vi "ScanBasic.vi"(8 "error in (no error)":errorcluster, 11 "data":variant[][](array[variant])) -> (0 "error out":errorcluster, 3 "Array":T1[](array[typedef]))   [LabVIEW 2017, in "Client.lvlib" / "ParserSorter.lvlib"]
doc: "Perform Basic Parsing"
uses:
  ParserSorter.lvlib
  SR Data.ctl
  AE Group.ctl
  SR Status.ctl
  SR Level.ctl
  SR Type.ctl
  <vilib>/addons/database/_DB Variant To Data/Database Variant To Data.xnode
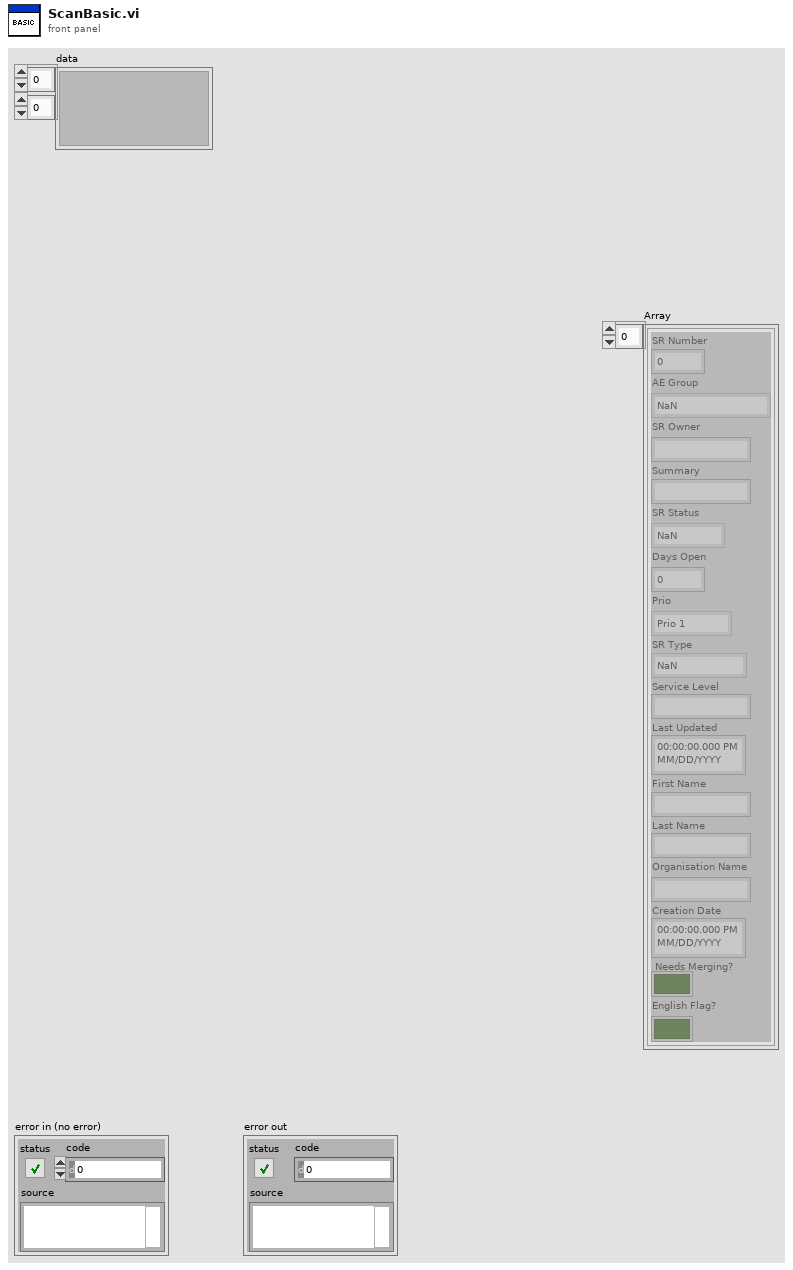
[diagram p1: front panel]
types:
  T1 = typedef "Client.lvlib/ParserSorter.lvlib/SR Data.ctl" = cluster{"SR Number":i64, "AE Group":T2, "SR Owner":string, "Summary":string, "SR Status":T3, "Days Open":dbl, "Prio":T4, "SR Type":T5, "Service Level":string, "Last Updated":timestamp, "First Name":string, "Last Name":string, "Organisation Name":string, "Creation Date":timestamp, "Needs Merging?":bool, "English Flag?":bool}
  T2 = typedef "Client.lvlib/ParserSorter.lvlib/AE Group.ctl" = enum32{"NaN", "AE-Germany", "AE-Poland", "AE-Switzerland", "AE-Czech Republic", "AE-Hungary", "AE-Romania", "AE-Slovakia", "AE-Slovenia"}
  T3 = typedef "Client.lvlib/ParserSorter.lvlib/SR Status.ctl" = enum32{"NaN", "Caller Abandoned", "Created in Error", "Declined to Purchase Support", "Expired", "Forum Resolved AE", "Forum Resolved Customer", "IN WORK", "IN WORK Collab with AES", "IN WORK Collab with PSE", "IN WORK Collab with SE", "IN WORK Escalation", "IN WORK Customer Added Note", "Open", "Potentially Resolved", "POC Resolved", "Resolved", "RMA Waiting on Customer", "RMA Open", "RMA In Progress", "RMA Closed - DOA", "RMA Closed", "RMA Approved for Return", "Project Complete", "Presumed Resolved", "IN WORK Wait on Customer"}
  T4 = typedef "Client.lvlib/ParserSorter.lvlib/SR Level.ctl" = enum16{"Prio 1", "Prio 2", "Prio 3", "Prio 4"}
  T5 = typedef "Client.lvlib/ParserSorter.lvlib/SR Type.ctl" = enum32{"NaN", "ATE Core Configurations (BYOATE)", "Activation", "BioBench", "CAN", "CM C Series", "Calibration", "Consulting Services", "CounterTimer", "DAQExpress", "DASYLab", "DIAdem", "DMM", "DSA HW", "Digital_IO", "FIRST (NIC Only)", "FieldBus", "FieldPoint", "Functional Savety", "GATI", "GPIB", "HMI and Industrial PCs", "HiQ", "HighSpeedDigital_IO", "IMAQ", "IOTech Vibration", "Industrial Communications", "InsightCM", "LV", "LV CD&Sim", "LV Comms", "LV Controls Add-Ons", "LV Embedded", "LV MathScript RT", "LV NXG", "LV NXT", "LVDSC", "LVFPGA", "LVPDA and LV Touch Panel", "LVRT", "LabWindows_CVI", "Lookout", "MATRIXx", "MStudioDotNet", "MStudioVisualBasic", "MStudioVisualC", "Measure (Legacy)", "Motion", "MultifunctionDAQ", "Multimedia Test HW/SW", "Multisim (EWB)", "NI Update Service", "OPC Servers", "Optical (OSI)", "PXI Controllers, Chassis, MXI", "PXI Timing and Sync", "Power Supplies and SMUs", "Powertrain Controls", "RAID", "RF", "RF Software", "RIO", "SC Express", "SCC", "SCXI", "SPEEDY-33 (Hyperception)", "STS", "ScopeDigitizers", "Serial", "Signal Sources", "SignalCondOther", "SignalExpress", "Software Defined Intruments", "Sound and Vibration SW", "Switch Executive", "Switches", "TestStand", "USRP", "Ultiboard (EWB)", "VBench", "VI Logger", "VXI_MXI", "VeriStand", "VisionSW", "VolumeLicenseMgr", "WSN", "Web UI Builder", "myRIO"}
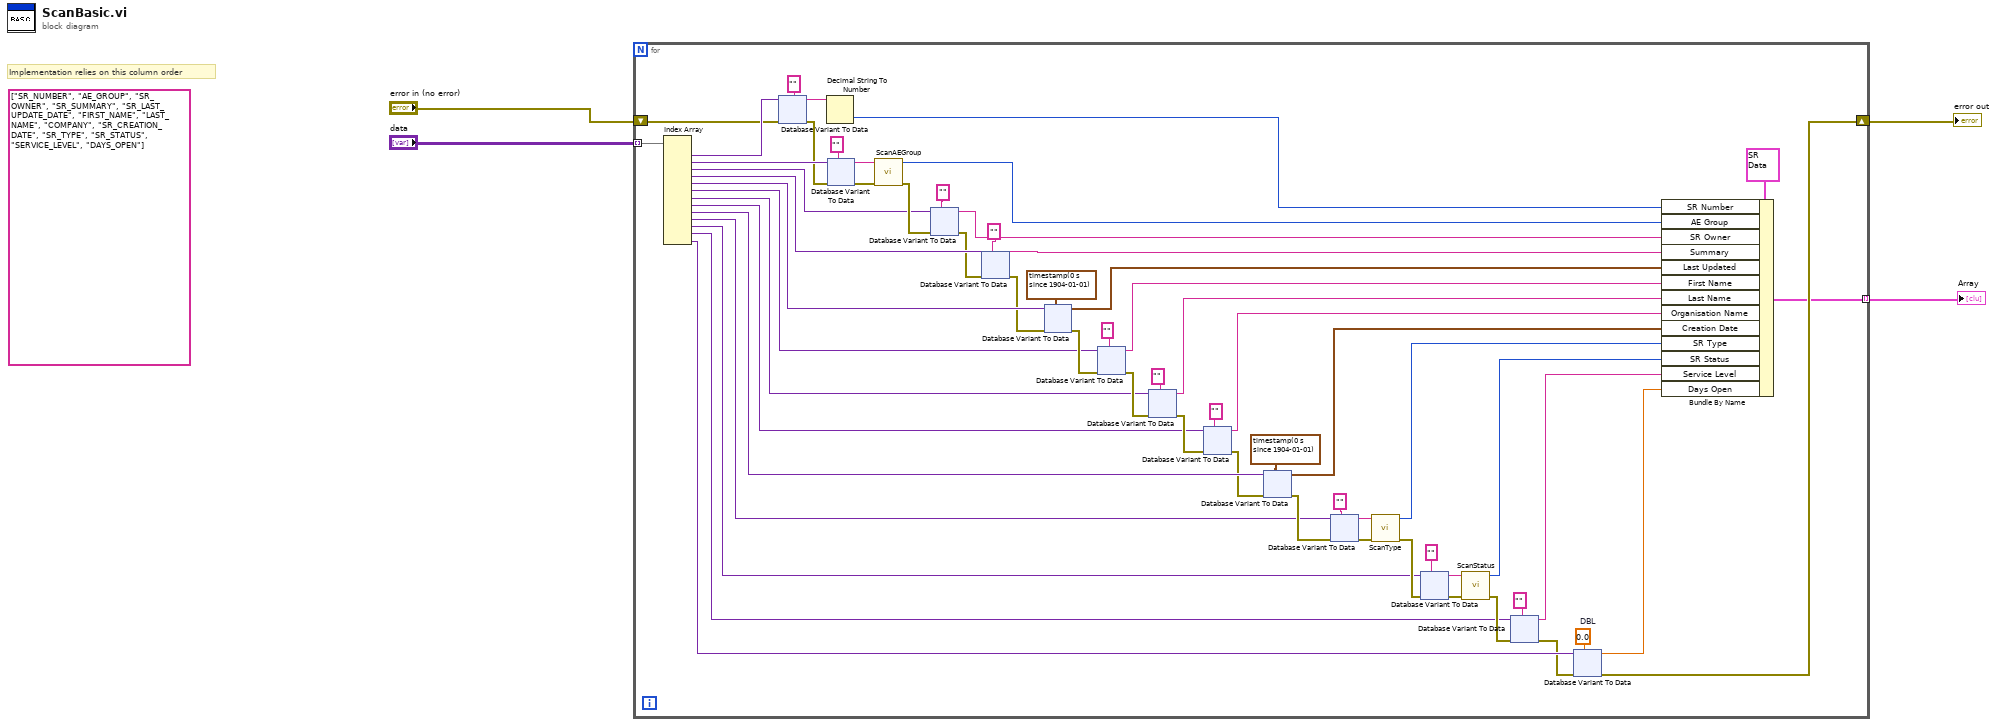
[diagram p0: block diagram]
diagram:
  (unwired) string[] ["SR_NUMBER", "AE_GROUP", "SR_OWNER", "SR_SUMMARY", "SR_LAST_UPDATE_DATE", "FIRST_NAME", "LAST_NAME", "COMPANY", "SR_CREATION_DATE", "SR_TYPE", "SR_STATUS", "SERVICE_LEVEL", "DAYS_OPEN"] ("appended array")
  # "Implementation relies on this column order"
  n1 = for {
    tunnel: "data" -> [w66] mode=indexing
    shift-right: [w7] -> w4
    shift-left: "error in (no error)" -> [w8]
    tunnel: [w6] -> w3 mode=indexing
    w10 = 0.0  # DBL
    n2 = Index Array(array=w66) -> (element #1=w65:variant, element #2=w62:variant, element #3=w54:variant, element #4=w51:variant, element #5=w48:variant, element #6=w40:variant, element #7=w39:variant, element #8=w34:variant, element #9=w32:variant, element #10=w27:variant, element #11=w18:variant, element #12=w15:variant, element #13=w12:variant)  [unwired: 13 in]
    n3 = xnode "Database Variant To Data"("database variant"=w65, "error in (no error)"=w8, "type"="" ("String")) -> ("data"=w64:string, "error out"=w61:errorcluster)
    n4 = Decimal String To Number(string=w64) -> (number=w5:i32)  [unwired: 2 in, 1 out]
    n5 = xnode "Database Variant To Data"("database variant"=w62, "error in (no error)"=w61, "type"="" ("String")) -> ("data"=w58:string, "error out"=w59:errorcluster)
    n6 = call "ScanAEGroup.vi"("error in (no error)"=w59, "AE Group String"=w58) -> ("error out"=w56:errorcluster, "AE Group"=w57:T2)  [unwired: 8 in]
    n7 = xnode "Database Variant To Data"("database variant"=w54, "error in (no error)"=w56, "type"="" ("String")) -> ("data"=w53:string, "error out"=w50:errorcluster)
    n8 = xnode "Database Variant To Data"("database variant"=w51, "error in (no error)"=w50, "type"="" ("String")) -> ("data"=w49:string, "error out"=w45:errorcluster)
    n9 = xnode "Database Variant To Data"("database variant"=w48, "error in (no error)"=w45, "type"=timestamp(0 s since 1904-01-01)) -> ("data"=w46:timestamp, "error out"=w44:errorcluster)
    n10 = xnode "Database Variant To Data"("database variant"=w40, "error in (no error)"=w44, "type"="" ("String")) -> ("data"=w38:string, "error out"=w43:errorcluster)
    n11 = xnode "Database Variant To Data"("database variant"=w39, "error in (no error)"=w43, "type"="" ("String")) -> ("data"=w37:string, "error out"=w36:errorcluster)
    n12 = xnode "Database Variant To Data"("database variant"=w34, "error in (no error)"=w36, "type"="" ("String")) -> ("data"=w33:string, "error out"=w30:errorcluster)
    n13 = xnode "Database Variant To Data"("database variant"=w32, "error in (no error)"=w30, "type"=timestamp(0 s since 1904-01-01)) -> ("data"=w29:timestamp, "error out"=w28:errorcluster)
    n14 = xnode "Database Variant To Data"("database variant"=w27, "error in (no error)"=w28, "type"="" ("String")) -> ("data"=w25:string, "error out"=w24:errorcluster)
    n15 = call "ScanType.vi"("error in (no error)"=w24, "Type String"=w25) -> ("error out"=w20:errorcluster, "SR Type"=w23:T5)  [unwired: 8 in]
    n16 = xnode "Database Variant To Data"("database variant"=w18, "error in (no error)"=w20, "type"="" ("String")) -> ("data"=w21:string, "error out"=w22:errorcluster)
    n17 = call "ScanStatus.vi"("error in (no error)"=w22, "Status String"=w21) -> ("error out"=w16:errorcluster, "SR Status"=w17:T3)  [unwired: 8 in]
    n18 = xnode "Database Variant To Data"("database variant"=w15, "error in (no error)"=w16, "type"="" ("String")) -> ("data"=w13:string, "error out"=w11:errorcluster)
    n19 = xnode "Database Variant To Data"("database variant"=w12, "error in (no error)"=w11, "type"=w10) -> ("data"=w9:dbl, "error out"=w7:errorcluster)
    n20 = Bundle By Name(cluster=T1 {"SR Number"=0, "AE Group"=enum."NaN", "SR Owner"="", "Summary"="", "SR Status"=enum."Open", "Days Open"=0.0, "Prio"=enum."Prio 1", "SR Type"=enum."OPC Servers", "Service Level"="", "Last Updated"=timestamp(0 s since 1904-01-01), "First Name"="", "Last Name"="", "Organisation Name"="", "Creation Date"=timestamp(0 s since 1904-01-01), "Needs Merging?"=FALSE, "English Flag?"=FALSE} ("SR Number"), "SR Number"=w5, "AE Group"=w57, "SR Owner"=w53, "Summary"=w49, "Last Updated"=w46, "First Name"=w38, "Last Name"=w37, "Organisation Name"=w33, "Creation Date"=w29, "SR Type"=w23, "SR Status"=w17, "Service Level"=w13, "Days Open"=w9) -> (w6:T1)
  }
  "error out" <- w4
  "Array" <- w3
